vi "CSM - List Modules.vi"(8 "Error In":errorcluster caption="error in (no error)", 9 "With Nodes? (F)":bool, 10 "Scope (Normal)":T1) -> (0 "error out":errorcluster, 3 "Module Names":string[](array[string]))   [LabVIEW 2017, in "Communicable State Machine.lvlib"]
doc: "### CSM - List Modules.vi\n\nList all active CSM modules.\n\n> [!NOTE] CSM Working Modes\n> 1. Stand-alone: Independent working mode. If no module name is provided, a random ID will be generated to identify the module.\n> 2. CSM: Regular CSM module.\n> 3. Action Worker: Worker mode. Add \"#\" after the module name to mark this module as a worker, sharing the same message queue with other workers of the same name.\n> 4. Chain Node: Chain node. Add \"$\" after the module name to mark this module as a chain node. Messages on the same chain will be passed sequentially until a node processes the message.\n\n\n-- <b>Controls</b> --\n- <b>Exclude Standalone CSM(T)</b>: Whether to include modules in standalone working mode\n\n-- <b>Indicators</b> --\n- <b>Module Names</b>: List of CSM module names"
uses:
  Communicable State Machine.lvlib
  _Support/Typedef/_CSM_List Module Scope.ctl
  _Support/CSMQ/_CSMOFGVOPER.ctl
  _Support/ChangeFlag/ChangeFlag-Read.vi
  _Support/ChangeFlag/ChangeFlagDB.vi
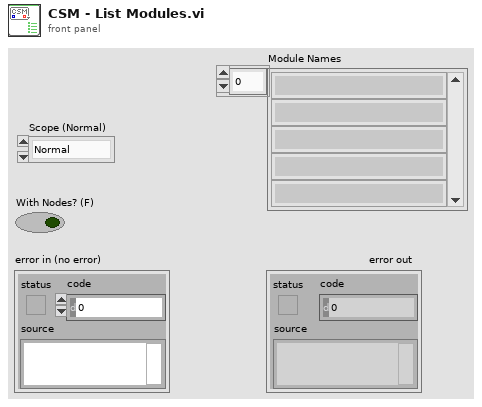
[diagram p1: front panel]
types:
  T1 = typedef "Communicable State Machine.lvlib/_CSM_List Module Scope.ctl" = enum16{"Normal", "System Only", "All"}
  T2 = typedef "Communicable State Machine.lvlib/_CSMOFGVOPER.ctl" = enum16{"Create If not Exist", "Get By Name", "List", "Check If Name Exists", "Release", "Module Status", "Create Status Event Handler", "Destroy Status Event Handler", "Clear Invalid Objs"}
  T3 = typedef "Communicable State Machine.lvlib/_CSMObj.ctl" = cluster{"info":T4, "Refs":T6}
  T4 = typedef "Communicable State Machine.lvlib/_CSMObj-Info.ctl" = cluster{"Module Name":string, "Requested Name":string, "Group Name":string, "Mode":T5, "Allowed Messages":string[]}
  T5 = typedef "Communicable State Machine.lvlib/_CSM_MODE.ctl" = enum16{"Not Exist", "Stand Alone", "CSM", "Worker", "Worker Agent", "Chain Node", "Chain"}
  T6 = typedef "Communicable State Machine.lvlib/_CSMObj-Refs.ctl" = cluster{"WatchDogQ":refnum<queue>, "CSMDataDVR":refnum<data-value>, "Queue":T7, "GroupDataDVR":refnum<data-value>, "TagMap":refnum<data-value>, "ExitEvent":refnum<user-event>, "NewStateEvent":refnum<user-event>, "StatusChangeEvent":refnum<user-event>}
  T7 = typedef "Communicable State Machine.lvlib/Priority Queue.ctl" = cluster{"HPriorityQ":refnum<queue>, "LowPriorityQ":refnum<queue>}
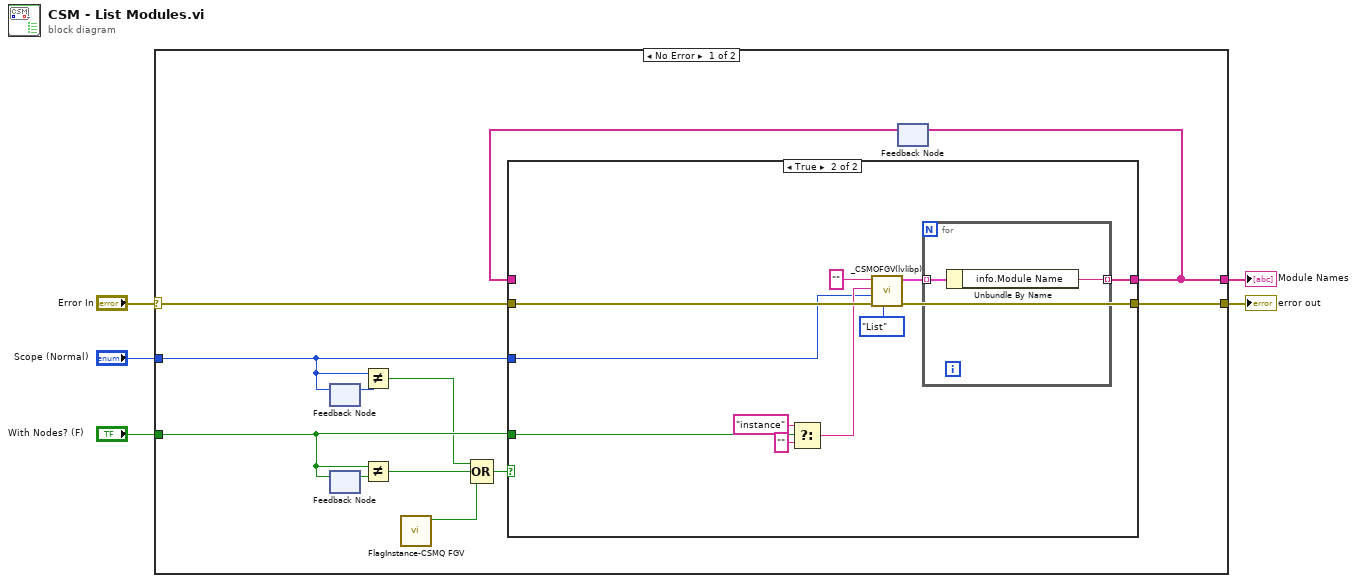
[diagram p0: block diagram]
diagram:
  n1 = case shown="No Error" "Error In" {
    selector: "Error In" -> [w17 w33]
    tunnel: [w16 w33] -> w4
    tunnel: "With Nodes? (F)" -> [w14 _]
    tunnel: [w10 _] -> w2
    tunnel: "Scope (Normal)" -> [w7 _]
    frame No Error {
      n2 = feedback #1() -> (w9:T1)  [unwired: 1 in]
      n3 = feedback-in #1(w7) -> ()
      n4 = feedback #2() -> (w15:bool)  [unwired: 1 in]
      n5 = feedback-in #2(w14) -> ()
      n6 = Not Equal?(x=w7, y=w9) -> (x != y?=w8:bool)
      n7 = Not Equal?(x=w14, y=w15) -> (x != y?=w13:bool)
      n8 = call "FlagInstance-CSMQ FGV.vi"() -> ("Changed"=w6:bool)  [unwired: 10 in, 1 out]
      n9 = Compound Arithmetic op=OR(w8, w13, w6) -> (w12:bool)
      n10 = feedback #3() -> (w11:string[])  [unwired: 1 in]
      n11 = case shown="True" w12 {
        tunnel: w17 -> [w19 w30]
        tunnel: [w19 w29] -> w16
        tunnel: w14 -> [_ w28]
        tunnel: [w18 w22] -> w10
        tunnel: w11 -> [w18 _]
        tunnel: w7 -> [_ w20]
        frame False {
        }
        frame True {
          n12 = Select(t="instance" ("Name (\"\" to Use UUID) in"), s=w28, f="" ("Name (\"\" to Use UUID) in")) -> (s? t:f=w21:string)
          n13 = call "_CSMOFGV(lvlibp).vi"("Operation"=_CSMOFGVOPER."List", "Error In"=w30, "Mode"=w20, "Reference"=w21, "Name (\"\" to Use UUID) In"="" ("Name (\"\" to Use UUID) in")) -> ("error out"=w29:errorcluster, "Array"=w23:T3[])  [unwired: 4 in, 1 out]
          n14 = for {
            tunnel: w23 -> [w32] mode=indexing
            tunnel: [w31] -> w22 mode=indexing
            n15 = Unbundle By Name(w32) -> ("info.Module Name"=w31:string)
          }
        }
      }
      n16 = feedback-in #3(w10) -> ()
    }
    frame Error {
    }
  }
  "error out" <- w4
  "Module Names" <- w2
